vi "add_MultiArrayLayout.vi"(5 "Data_Offset":u32, 6 "Array":T1, 7 "msg in":string) -> (3 "msg out":string)   [LabVIEW 2012]
doc: "Flattens a multi array layout into a message"
uses:
  <userlib>/ROS for LabVIEW Software/ROS/MessageBuilding/std_msgs/subs/u32Scalar.vi
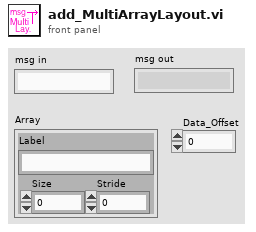
[diagram p1: front panel]
types:
  T1 = cluster{"Label":string, "Size":u32, "Stride":u32}
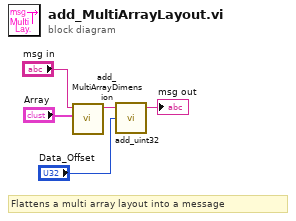
[diagram p0: block diagram]
diagram:
  # "Flattens a multi array layout into a message"
  n1 = call <userlib>:"add_MultiArrayDimension.vi"("Array"="Array", "msg in"="msg in") -> ("msg out"=w1:string)  [unwired: 5 in]
  n2 = call-poly <userlib>:"add_uint32.vi"("Numeric"="Data_Offset", "msg in"=w1) -> ("msg out"=→"msg out":string)  [unwired: 3 in]
